vi "FreddysMontyHall.vi"() -> ()   [LabVIEW 2026]
panel:
  out "DOOR 10":bool
  out "DOOR 9":bool
  out "DOOR 8":bool
  out "DOOR 7":bool
  out "DOOR 6":bool
  out "DOOR 5":bool
  out "DOOR 4":bool
  out "Blood":bool
  out "Success Rate %":i32
  out "Freddy Found":i32
  out "Number of Games":i32
  in  "User pick":T1
  out "Win?":bool
  in  "?":bool
  in  "Stay":bool
  in  "Switch":bool
  out "DOOR 3":bool
  out "DOOR 2":bool
  out "DOOR 1":bool
  out "Instructions and Introduction":string
  in  "?":bool
  out "?":T2
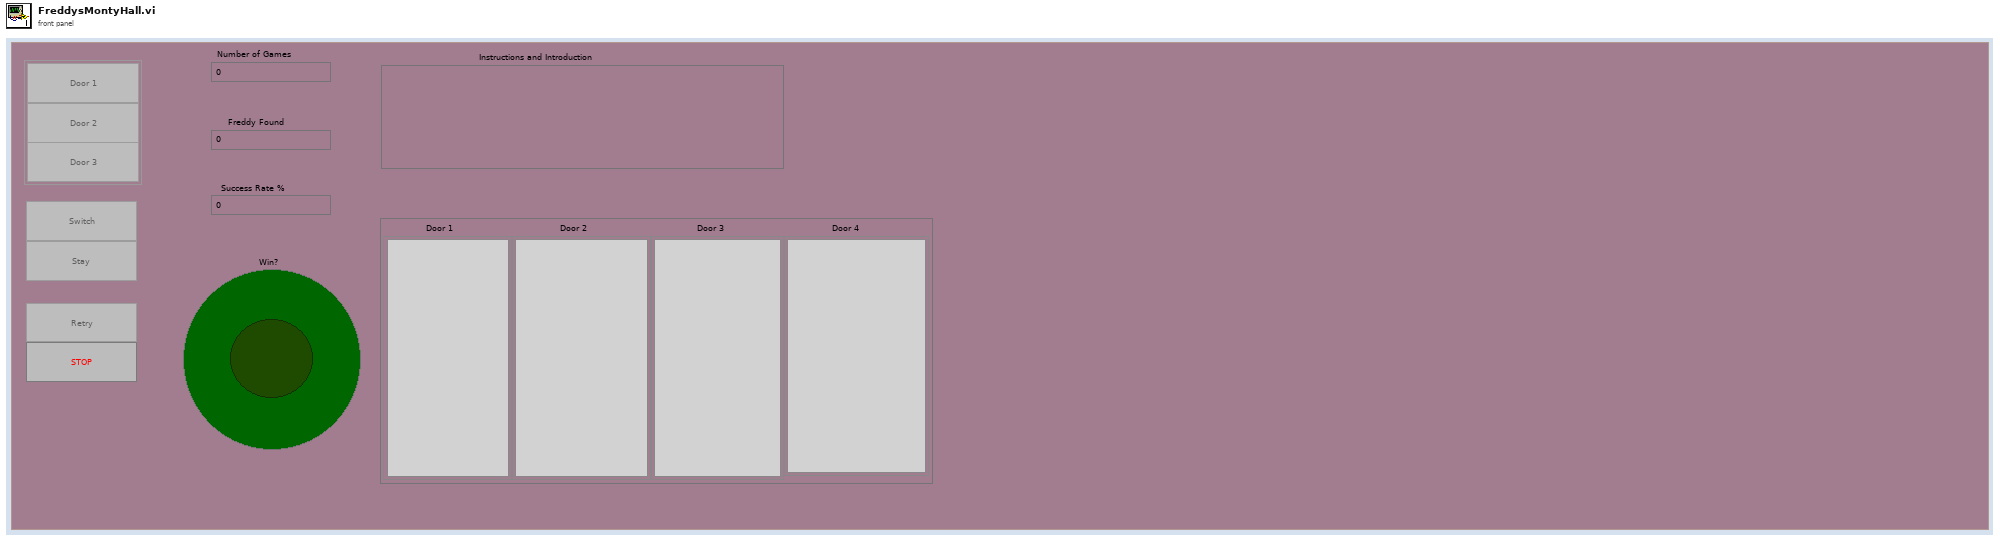
[diagram p1: front panel]
types:
  T1 = cluster{"Switch 2":bool, "Stay 2":bool, "Stay 3":bool}
  T2 = cluster{"Door 1":u16, "Door 2":u16, "Door 3":u16, "Door 4":u16}
  T3 = enum16{"start", "Make", "choose", "swap", "show", "result"}
  T4 = cluster{"open":bool[], "player":bool[], "result":bool, "freddy":i32, "playerpickeddoor\n":i32, "second":i32, "playercur":i32, "dooropen":cluster{"[0]":u16, "[1]":u16, "[2]":u16, i32}, "games":i32, "wins":i32}
  T5 = enum8{"Enabled", "Disabled", "Disabled and Grayed Out"}
  T6 = cluster{"[0]":u16, "[1]":u16, "[2]":u16, "[3]":u16}
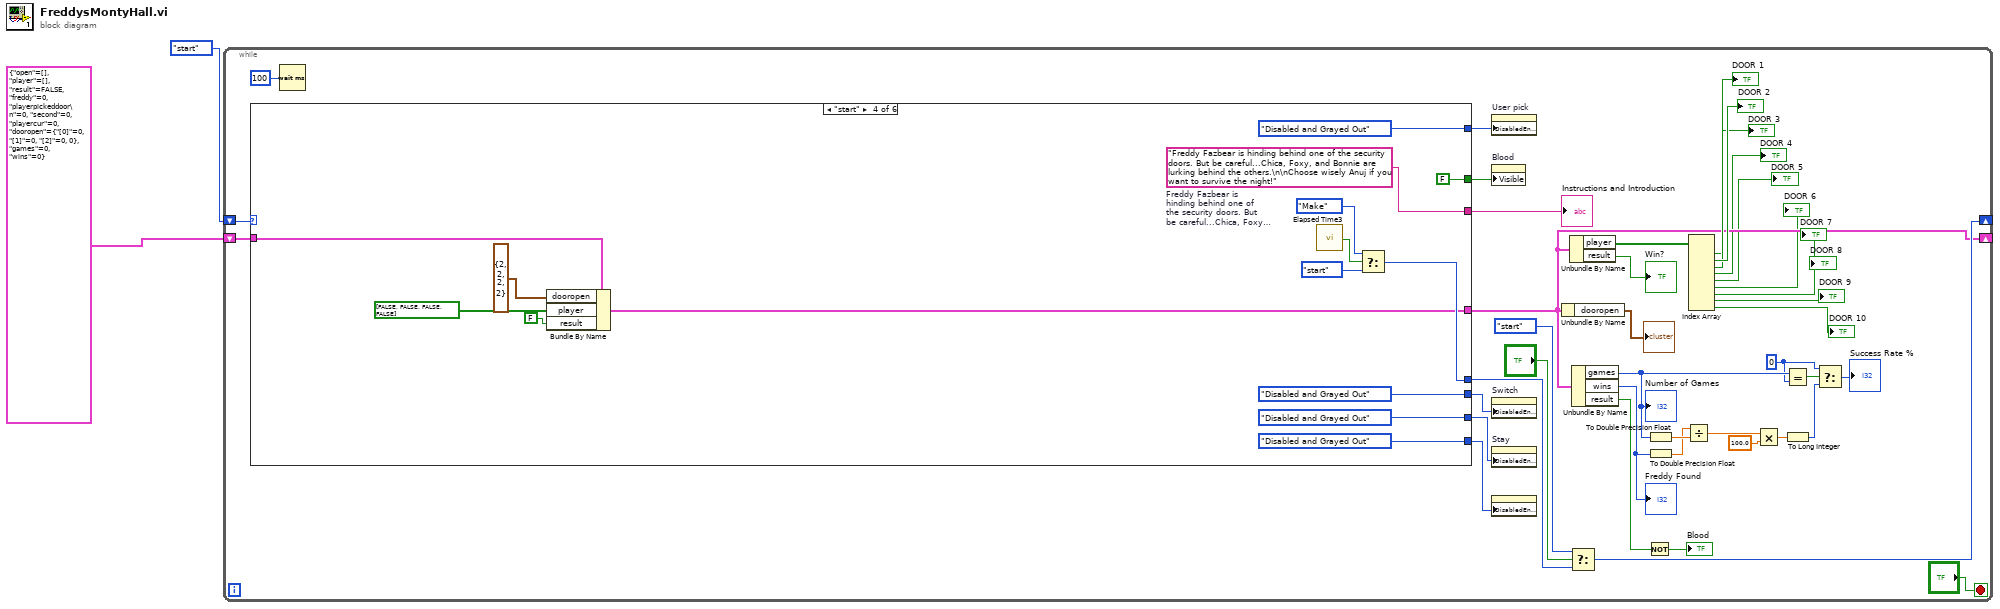
[diagram p0: block diagram]
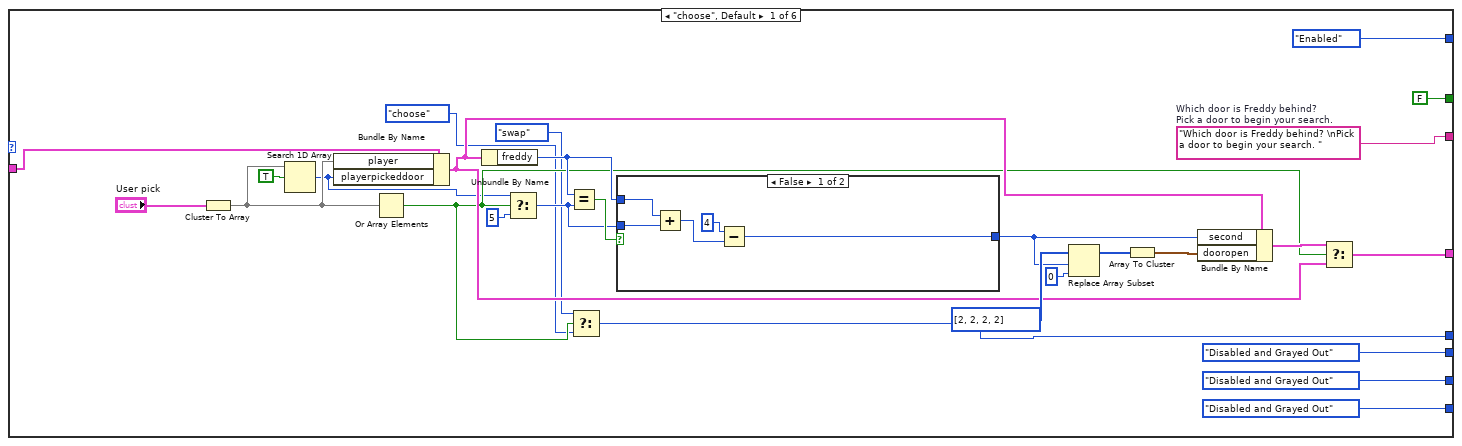
[diagram p2: hidden frame]
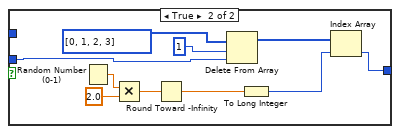
[diagram p3: hidden frame]
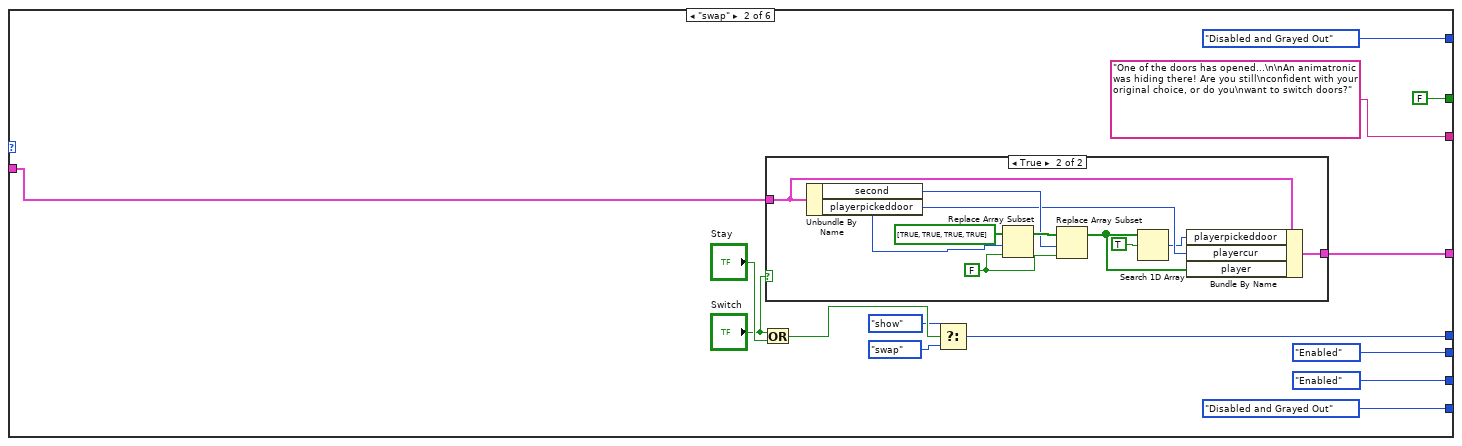
[diagram p4: hidden frame]
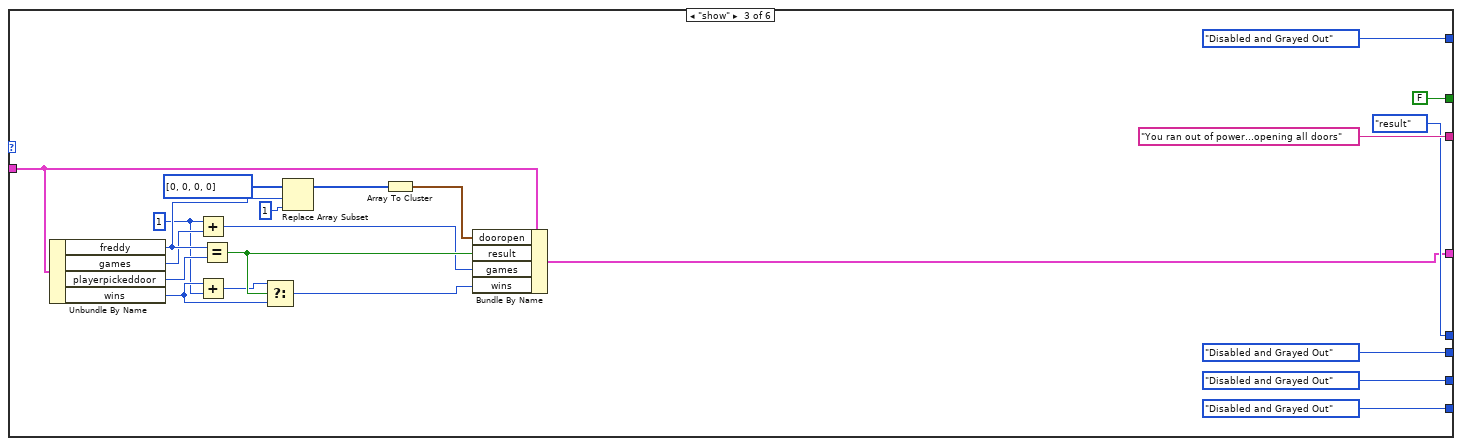
[diagram p6: hidden frame]
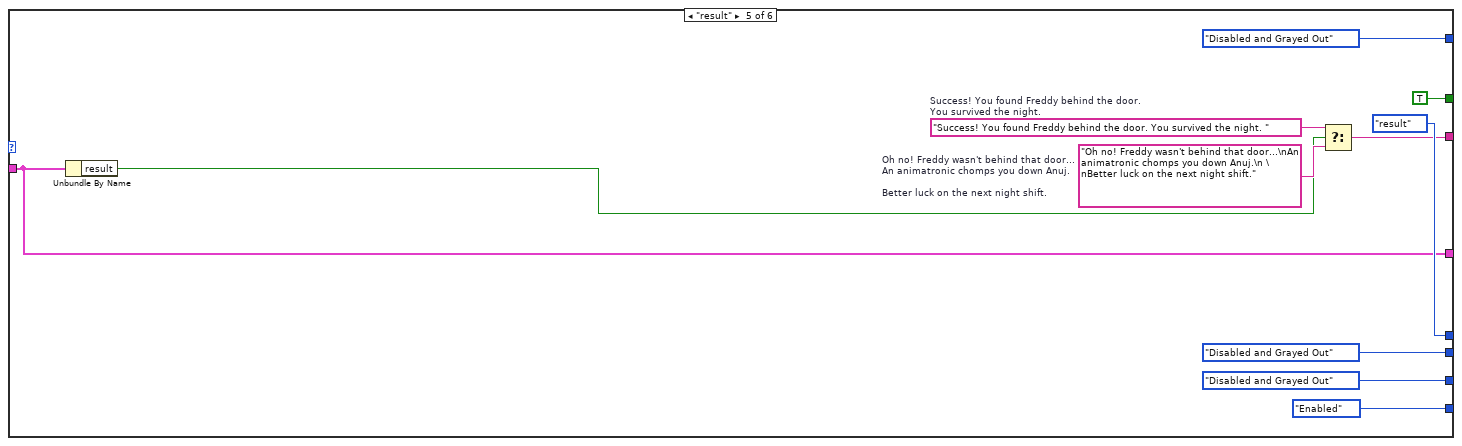
[diagram p7: hidden frame]
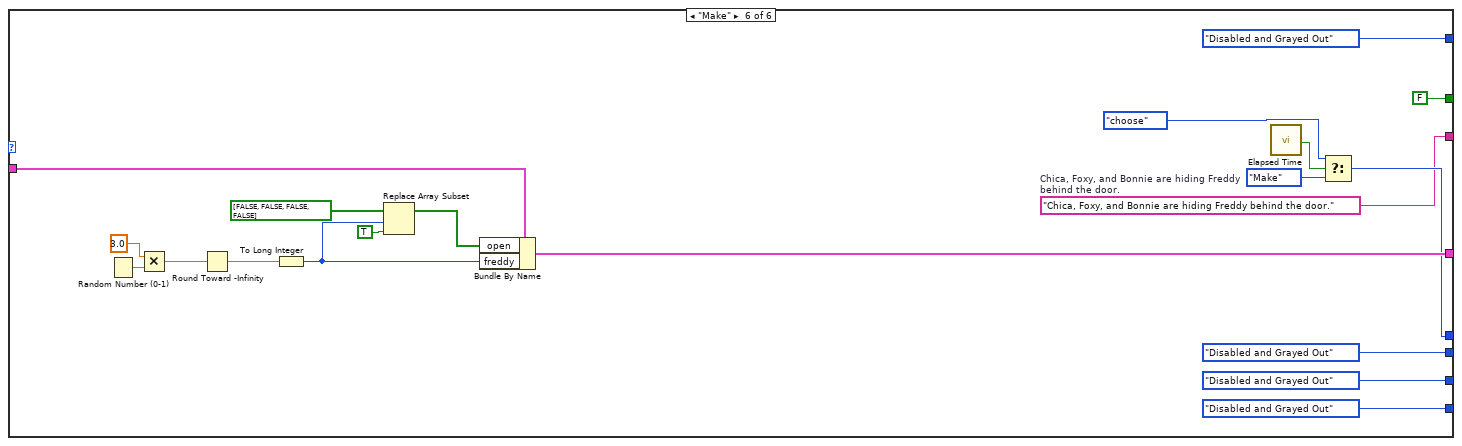
[diagram p8: hidden frame]
diagram:
  n1 = while {
    shift-right: [w31] -> _
    shift-left: T3."start" -> [w39]
    shift-right: [w10] -> _
    shift-left: T4 {"open"=[], "player"=[], "result"=FALSE, "freddy"=0, "playerpickeddoor\n"=0, "second"=0, "playercur"=0, "dooropen"={"[0]"=0, "[1]"=0, "[2]"=0, 0}, "games"=0, "wins"=0} -> [w40]
    stop <- "?" stop-if-true
    w11 = 0
    n2 = case shown="\"start\"" w39 {
      tunnel: w40 -> [w69 w90 w124 w142 w149 w172]
      tunnel: [w55 w89 w126 w143 w149 w170] -> w10
      tunnel: [w59 w94 T3."result" w144 T3."result" w169] -> w32
      tunnel: [w68 "One of the doors has opened...\n\nAn animatronic was hiding there! Are you still\nconfident with your original choice, or do you\nwant to switch doors?" "You ran out of power...opening all doors" w146 w150 w167] -> w38
      tunnel: [T5."Enabled" ("Disabled") T5."Disabled and Grayed Out" ("Disabled") T5."Disabled and Grayed Out" ("Disabled") T5."Disabled and Grayed Out" ("Disabled") T5."Disabled and Grayed Out" ("Disabled") T5."Disabled and Grayed Out" ("Disabled")] -> w28
      tunnel: [T5."Disabled and Grayed Out" ("Disabled") T5."Enabled" ("Disabled") T5."Disabled and Grayed Out" ("Disabled") T5."Disabled and Grayed Out" ("Disabled") T5."Disabled and Grayed Out" ("Disabled") T5."Disabled and Grayed Out" ("Disabled")] -> w27
      tunnel: [T5."Disabled and Grayed Out" ("Disabled") T5."Enabled" ("Disabled") T5."Disabled and Grayed Out" ("Disabled") T5."Disabled and Grayed Out" ("Disabled") T5."Disabled and Grayed Out" ("Disabled") T5."Disabled and Grayed Out" ("Disabled")] -> w26
      tunnel: [T5."Disabled and Grayed Out" ("Disabled") T5."Disabled and Grayed Out" ("Disabled") T5."Disabled and Grayed Out" ("Disabled") T5."Disabled and Grayed Out" ("Disabled") T5."Enabled" ("Disabled") T5."Disabled and Grayed Out" ("Disabled")] -> w25
      tunnel: [FALSE ("Visible") FALSE ("Visible") FALSE ("Visible") FALSE ("Visible") TRUE ("Visible") FALSE ("Visible")] -> w16
      frame "choose", Default {
        w68 = "Which door is Freddy behind? \nPick a door to begin your search. "  # Which door is Freddy behind?  Pick a door to begin your search.
        n3 = Cluster To Array(cluster="User pick") -> (array=w66:bool[])
        n4 = Search 1D Array(1D array=w66, element=TRUE) -> (index of element=w52:i32)  [unwired: 1 in]
        n5 = Bundle By Name(cluster=w69, "player"=w66, "playerpickeddoor"=w52) -> (w57:T4)
        n6 = Or Array Elements(Boolean array=w66) -> (logical OR=w54:bool)
        n7 = Unbundle By Name(w57) -> ("freddy"=w60:i32)
        n8 = Select(t=w52, s=w54, f=5 ("length")) -> (s? t:f=w53:i32)
        n9 = Equal?(x=w60, y=w53) -> (x = y?=w61:bool)
        n10 = Select(t=T3."swap", s=w54, f=T3."choose") -> (s? t:f=w59:T3)
        n11 = case shown="False" w61 {
          tunnel: w53 -> [w72 w78]
          tunnel: w60 -> [w71 _]
          tunnel: [w70 w75] -> w58
          frame False {
            n12 = Add(x=w71, y=w72) -> (x+y=w74:i32)
            n13 = Subtract(x=4, y=w74) -> (x-y=w70:i32)
          }
          frame True {
            n14 = Random Number (0-1)() -> (number: 0 to 1=w81:dbl)
            n15 = Multiply(x=w81, y=2.0) -> (x*y=w83:dbl)
            n16 = Round Toward -Infinity(1:w83) -> (0:w80:dbl)
            n17 = Delete From Array(array=i32[] [0, 1, 2, 3], length=1, index=w78) -> (array with subset deleted=w76:i32[])  [unwired: 1 out]
            n18 = To Long Integer(number=w80) -> (32bit integer=w77:i32)
            n19 = Index Array(array=w76, index=w77) -> (element=w75:i32)
          }
        }
        n20 = Replace Array Subset(array=u16[] [2, 2, 2, 2], new element=u16 0 ("new element/subarray"), index=w58) -> (w64:u16[])
        n21 = Array To Cluster(array=w64) -> (cluster=w43:T6)
        n22 = Bundle By Name(cluster=w57, "second"=w58, "dooropen"=w43) -> (w56:T4)
        n23 = Select(t=w56, s=w54, f=w57) -> (s? t:f=w55:T4)
      }
      frame "swap" {
        n24 = Or(x="Switch", y="Stay") -> (x .or. y?=w95:bool)
        n25 = case shown="True" "Switch" {
          tunnel: w90 -> [w99 w109]
          tunnel: [w99 w108] -> w89
          frame False {
          }
          frame True {
            w102 = FALSE
            n26 = Unbundle By Name(w109) -> ("second"=w105:i32, "playerpickeddoor"=w104:i32)
            n27 = Replace Array Subset(array=bool[] [TRUE, TRUE, TRUE, TRUE], new element=w102, index=w104) -> (w106:bool[])
            n28 = Replace Array Subset(array=w106, new element=w102, index=w105) -> (w103:bool[])
            n29 = Search 1D Array(1D array=w103, element=TRUE) -> (index of element=w101:i32)  [unwired: 1 in]
            n30 = Bundle By Name(cluster=w109, "playerpickeddoor"=w101, "playercur"=w104, "player"=w103) -> (w108:T4)
          }
        }
        n31 = Select(t=T3."show", s=w95, f=T3."swap") -> (s? t:f=w94:T3)
      }
      frame "show" {
        w112 = 1
        n32 = Unbundle By Name(w124) -> ("freddy"=w122:i32, "games"=w117:i32, "playerpickeddoor"=w123:i32, "wins"=w113:i32)
        n33 = Add(x=w112, y=w117) -> (x+y=w115:i32)
        n34 = Add(x=w113, y=w112) -> (x+y=w111:i32)
        n35 = Equal?(x=w122, y=w123) -> (x = y?=w118:bool)
        n36 = Select(t=w111, s=w118, f=w113) -> (s? t:f=w114:i32)
        n37 = Replace Array Subset(array=u16[] [0, 0, 0, 0], new element=u16 1 ("new element/subarray"), index=w122) -> (w128:u16[])
        n38 = Array To Cluster(array=w128) -> (cluster=w125:T6)
        n39 = Bundle By Name(cluster=w124, "dooropen"=w125, "result"=w118, "games"=w115, "wins"=w114) -> (w126:T4)
      }
      frame "start" {
        w146 = "Freddy Fazbear is hinding behind one of the security doors. But be careful...Chica, Foxy, and Bonnie are lurking behind the others.\n\nChoose wisely Anuj if you want to survive the night!"  # Freddy Fazbear is hinding behind one of the security doors. But be careful...Chica, Foxy, and Bonnie are lurking behind the others.  Choose wisely Anuj if you want to survive the night!
        n40 = Bundle By Name(cluster=w142, "dooropen"=cluster{"[0]":u16, "[1]":u16, "[2]":u16, i32} {"[0]"=2, "[1]"=2, "[2]"=2, 2}, "player"=bool[] [FALSE, FALSE, FALSE, FALSE], "result"=FALSE) -> (w143:T4)
        n41 = call "Elapsed Time3"() -> ("Time has Elapsed"=w145:bool)  [unwired: 12 in, 7 out]
        n42 = Select(t=T3."Make", s=w145, f=T3."start") -> (s? t:f=w144:T3)
      }
      frame "result" {
        w152 = "Oh no! Freddy wasn't behind that door...\nAn animatronic chomps you down Anuj.\n \nBetter luck on the next night shift."  # Oh no! Freddy wasn't behind that door... An animatronic chomps you down Anuj.   Better luck on the next night shift.
        w151 = "Success! You found Freddy behind the door. You survived the night. "  # Success! You found Freddy behind the door. You survived the night.
        n43 = Unbundle By Name(w149) -> ("result"=w148:bool)
        n44 = Select(t=w151, s=w148, f=w152) -> (s? t:f=w150:string)
      }
      frame "Make" {
        w167 = "Chica, Foxy, and Bonnie are hiding Freddy behind the door."  # Chica, Foxy, and Bonnie are hiding Freddy behind the door.
        n45 = Random Number (0-1)() -> (number: 0 to 1=w176:dbl)
        n46 = Multiply(x=3.0, y=w176) -> (x*y=w175:dbl)
        n47 = Round Toward -Infinity(1:w175) -> (0:w162:dbl)
        n48 = To Long Integer(number=w162) -> (32bit integer=w163:i32)
        n49 = Replace Array Subset(array=bool[] [FALSE, FALSE, FALSE, FALSE], new element=TRUE, index=w163) -> (w171:bool[])
        n50 = Bundle By Name(cluster=w172, "open"=w171, "freddy"=w163) -> (w170:T4)
        n51 = call "Elapsed Time"() -> ("Time has Elapsed"=w168:bool)  [unwired: 12 in, 7 out]
        n52 = Select(t=T3."choose", s=w168, f=T3."Make") -> (s? t:f=w169:T3)
      }
    }
    "Instructions and Introduction" <- w38
    n53 = Wait (ms)(milliseconds to wait=u32 100) -> ()  [unwired: 1 out]
    n54 = property on="User pick" class="Clust"("DisabledEnum"=w28) -> ()  [unwired: 2 in, 2 out]
    n55 = property on="Blood" class="Bool (strict)"("Visible"=w16) -> ()  [unwired: 2 in, 2 out]
    n56 = property on="Switch" class="Bool"("DisabledEnum"=w27) -> ()  [unwired: 2 in, 2 out]
    n57 = property on="Stay" class="Bool"("DisabledEnum"=w26) -> ()  [unwired: 2 in, 2 out]
    n58 = property class="Bool"("DisabledEnum"=w25) -> ()  [unwired: 2 in, 2 out]
    n59 = Unbundle By Name(w10) -> ("dooropen"=→"?":cluster{"[0]":u16, "[1]":u16, "[2]":u16, i32})
    n60 = Unbundle By Name(w10) -> ("player"=w36:bool[], "result"=→"Win?":bool)
    n61 = Select(t=T3."start", s="?", f=w32) -> (s? t:f=w31:T3)
    n62 = Unbundle By Name(w10) -> ("games"=w15:i32, "wins"=w20:i32, "result"=w17:bool)
    "Number of Games" <- w15
    "Freddy Found" <- w20
    n63 = Not(x=w17) -> (.not. x?=→"Blood":bool)
    n64 = To Double Precision Float(number=w15) -> (double precision float=w22:dbl)
    n65 = To Double Precision Float(number=w20) -> (double precision float=w21:dbl)
    n66 = Divide(x=w21, y=w22) -> (x/y=w23:dbl)
    n67 = Index Array(array=w36) -> (element #1=→"DOOR 1":bool, element #2=→"DOOR 2":bool, element #3=→"DOOR 3":bool, element #4=→"DOOR 4":bool, element #5=→"DOOR 5":bool, element #6=→"DOOR 6":bool, element #7=→"DOOR 7":bool, element #8=→"DOOR 9":bool, element #9=→"DOOR 10":bool)  [unwired: 9 in]
    n68 = Multiply(x=w23, y=100.0) -> (x*y=w24:dbl)
    n69 = Equal?(x=w15, y=w11) -> (x = y?=w12:bool)
    n70 = To Long Integer(number=w24) -> (32bit integer=w13:i32)
    n71 = Select(t=w11, s=w12, f=w13) -> (s? t:f=→"Success Rate %":i32)
  }
